vi "ReportProcess.vi"(8 "error in":errorcluster caption="错误输入（无错误）", 10 "text data":string[][](array[string]), 11 "Path":path caption="模板（空）") -> (0 "error out":errorcluster caption="错误输出")   [LabVIEW 2013]
uses:
  <vilib>/Utility/NIReport.llb/NI_report.lvclass
  <vilib>/addons/_office/_exclsub.llb/font.ctl
  <vilib>/Utility/NIReport.llb/Append Text Table to Report (wrap).vi
  <vilib>/addons/_office/excel.llb/Excel Easy Table (str).vi
  <vilib>/Utility/NIReport.llb/Excel/NI_Excel.lvclass
  <vilib>/addons/_office/NI_ReportGenerationToolkit.lvlib
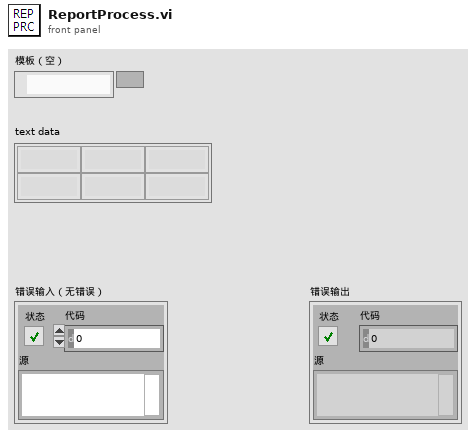
[diagram p1: front panel]
types:
  T1 = enum16{"maximized", "minimized", "normal", "no change"}
  T2 = enum16{"Standard Report", "HTML", "Word", "Excel"}
  T3 = typedef "NI_ReportGenerationToolkit.lvlib/font.ctl" = cluster{"font name":string, "font size":dbl, "bold":u16, "italic":u16, "underline":u16, "strike through":u16, "font color":u32}
  T4 = cluster{"position (Excel)":cluster{"row":i32, "column":i32}, "name (Excel)":string, "bookmark (Word)":string}
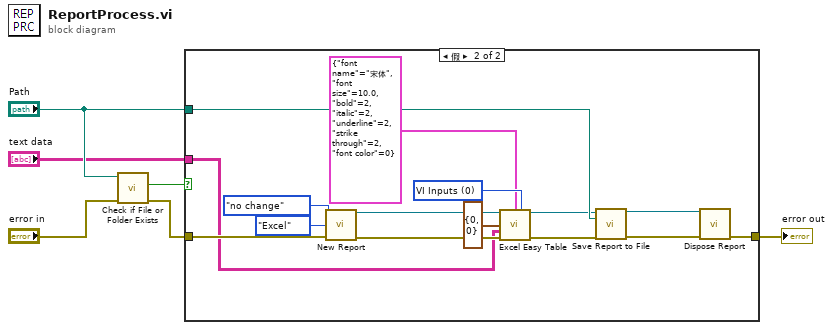
[diagram p0: block diagram]
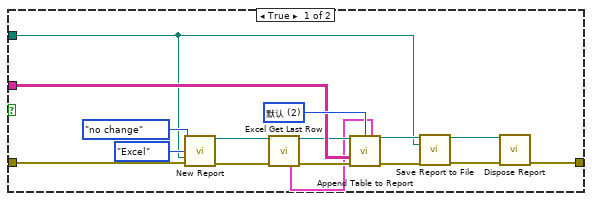
[diagram p2: hidden frame]
diagram:
  n1 = call <vilib>:"Check if File or Folder Exists.vi"("error in (no error)"="error in", "path"="Path") -> ("error out"=w2:errorcluster, "file or folder exists?"=w4:bool)  [unwired: 7 in, 1 out]
  n2 = case shown="假" w4 {
    tunnel: [w17 w34] -> w6
    tunnel: "Path" -> [w7 w32]
    tunnel: w2 -> [w14 w31]
    tunnel: "text data" -> [w13 w23]
    frame True {
      w15 = u16 2 items=["US", "公制", "默认"] ("measurement system")
      n3 = call <vilib>:"New Report.vi"("window state (normal)"=T1."no change", "report type"=T2."Excel", "template (empty)"=w7, "error in (no error)"=w14) -> ("report out"=w12:refnum<class "NI_report.lvclass">, "error out"=w10:errorcluster)  [unwired: 10 in]
      n4 = call <vilib>:"Excel Get Last Row.vi"("report in"=w12, "error in (no error)"=w10) -> ("report out"=w11:refnum<class "NI_report.lvclass">, "MS Office parameters out"=w8:T4, "error out"=w9:errorcluster)  [unwired: 11 in]
      n5 = call-poly <vilib>:"Append Table to Report.vi"("report in"=w11, "measurement system"=w15, "MS Office parameters"=w8, "text data"=w13, "error in (no error)"=w9) -> ("report out"=w21:refnum<class "NI_report.lvclass">, "error out"=w20:errorcluster)  [unwired: 7 in, 2 out]
      n6 = call-dynamic "Save Report to File.vi"("report in"=w21, "report file path"=w7, "error in (no error)"=w20) -> ("report out"=w19:refnum<class "NI_report.lvclass">, "error out"=w18:errorcluster)  [unwired: 11 in]
      n7 = call-dynamic "Dispose Report.vi"("report in"=w19, "error in (no error)"=w18) -> ("error out"=w17:errorcluster)  [unwired: 13 in]
    }
    frame False {
      w26 = u16 0 items=["VI Inputs", "Font Dialog Box"] ("font settings source")
      n8 = call <vilib>:"New Report.vi"("window state (normal)"=T1."no change", "report type"=T2."Excel", "error in (no error)"=w31) -> ("report out"=w30:refnum<class "NI_report.lvclass">, "error out"=w28:errorcluster)  [unwired: 11 in]
      n9 = call-poly <vilib>:"Excel Easy Table.vi"("report in"=w30, "font"=T3 {"font name"="宋体", "font size"=10.0, "bold"=2, "italic"=2, "underline"=2, "strike through"=2, "font color"=0}, "font settings source"=w26, "start (0, 0)"=cluster{"row":i32, "column":i32} {"row"=0, "column"=0}, "text data"=w23, "error in (no error)"=w28) -> ("report out"=w29:refnum<class "NI_report.lvclass">, "error out"=w27:errorcluster)  [unwired: 5 in, 3 out]
      n10 = call-dynamic "Save Report to File.vi"("report in"=w29, "report file path"=w32, "error in (no error)"=w27) -> ("report out"=w36:refnum<class "NI_report.lvclass">, "error out"=w35:errorcluster)  [unwired: 11 in]
      n11 = call-dynamic "Dispose Report.vi"("report in"=w36, "error in (no error)"=w35) -> ("error out"=w34:errorcluster)  [unwired: 13 in]
    }
  }
  "error out" <- w6
